vi "Insitu_y-data modification.vi"(9 "length":i32, 10 "index":i32, 11 "all data":dbl[][](array[numeric])) -> (3 "output":dbl[](array[numeric]))   [LabVIEW 2020]
panel:
  in  "menu":enum16{"Subtraction"}(ring)
  in  "col2":i32
  in  "col 1":i32
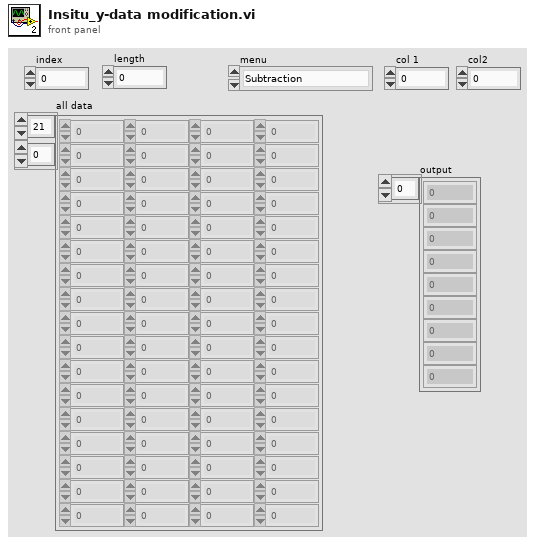
[diagram p1: front panel]
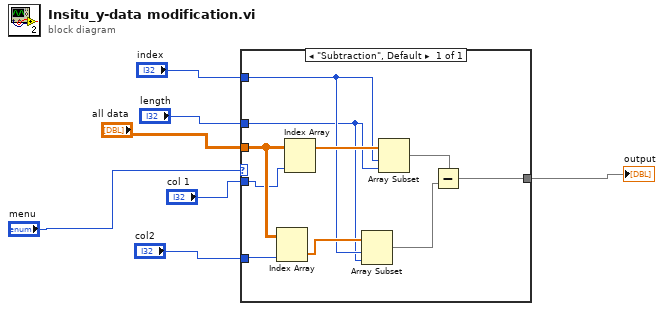
[diagram p0: block diagram]
diagram:
  n1 = case shown="\"Subtraction\", Default" "menu" {
    tunnel: "col 1" -> [w9]
    tunnel: "all data" -> [w17]
    tunnel: "col2" -> [w8]
    tunnel: [w16] -> w4
    tunnel: "index" -> [w13]
    tunnel: "length" -> [w12]
    frame "Subtraction", Default {
      n2 = Index Array(array=w17, index (col)=w8) -> (element=w14:dbl[])  [unwired: 1 in]
      n3 = Index Array(array=w17, index (col)=w9) -> (element=w15:dbl[])  [unwired: 1 in]
      n4 = Array Subset(array=w14, index=w13, length=w12) -> (w10:dbl[])
      n5 = Array Subset(array=w15, index=w13, length=w12) -> (w11:dbl[])
      n6 = Subtract(x=w11, y=w10) -> (x-y=w16:dbl[])
    }
  }
  "output" <- w4
